vi "内置参数设置.vi"() -> ()   [LabVIEW 2016, in "斯坦道CODMn新电路板.lvlib"]
uses:
  <vilib>/Utility/miscctls.llb/LVPointTypeDef.ctl
panel:
  in  "阀配置:":u8(ring) items=["三通阀", "排阀"]
  in  "AB跨度告警值:":u16
  in  "B值告警上限值:":u16
  in  "B值范围:":u16
  in  "A值告警上限值:":u16
  in  "A值范围:":u16
  in  "是否存在液位检测板:":u16(ring) items=["否", "是"]
  in  "检出限(mg/L):":dbl
  in  "测量精度(mg/L):":dbl
  in  "ILimitDown":dbl
  in  "ILimitUp:":dbl
  in  "K d:":dbl
  in  "K i:":dbl
  in  "K p:":dbl
  in  "加热超时时间:(单位:秒)":dbl
  in  "告警温度:":dbl
  in  "加热温度:  校准参数":dbl
  in  "运行速度:  (修改需要重启)":u16
  in  "偏心轮: 校准参数":dbl
  in  "注射泵加热超时时间(s):":u16
  in  "注射泵保温温度H:":u8
  in  "注射泵\n保温温度L:":u8
  in  "废液通道:":u8
  in  "纯水通道:":u8
  in  "滴定速度:":u16
  in  "出样速度:":u16
  in  "进样速度:":u16
  in  "阀数量:":u8(ring) items=["9通"=9, "12通"=12]
  in  "注射泵型号":u8(ring) items=["TECAN", "润泽"]
  in  "阈值(高→低)(mg/L):":dbl
  in  "阈值(低→高)(mg/L):":dbl
  in  "检测下限(mg/L):":dbl
  in  "检测上限(mg/L):":dbl
  in  "关闭":bool
  in  "保存":bool
  in  "读取":bool
  # "仪器内部参数设置"
  # "~"
  # "~"
  # "~"
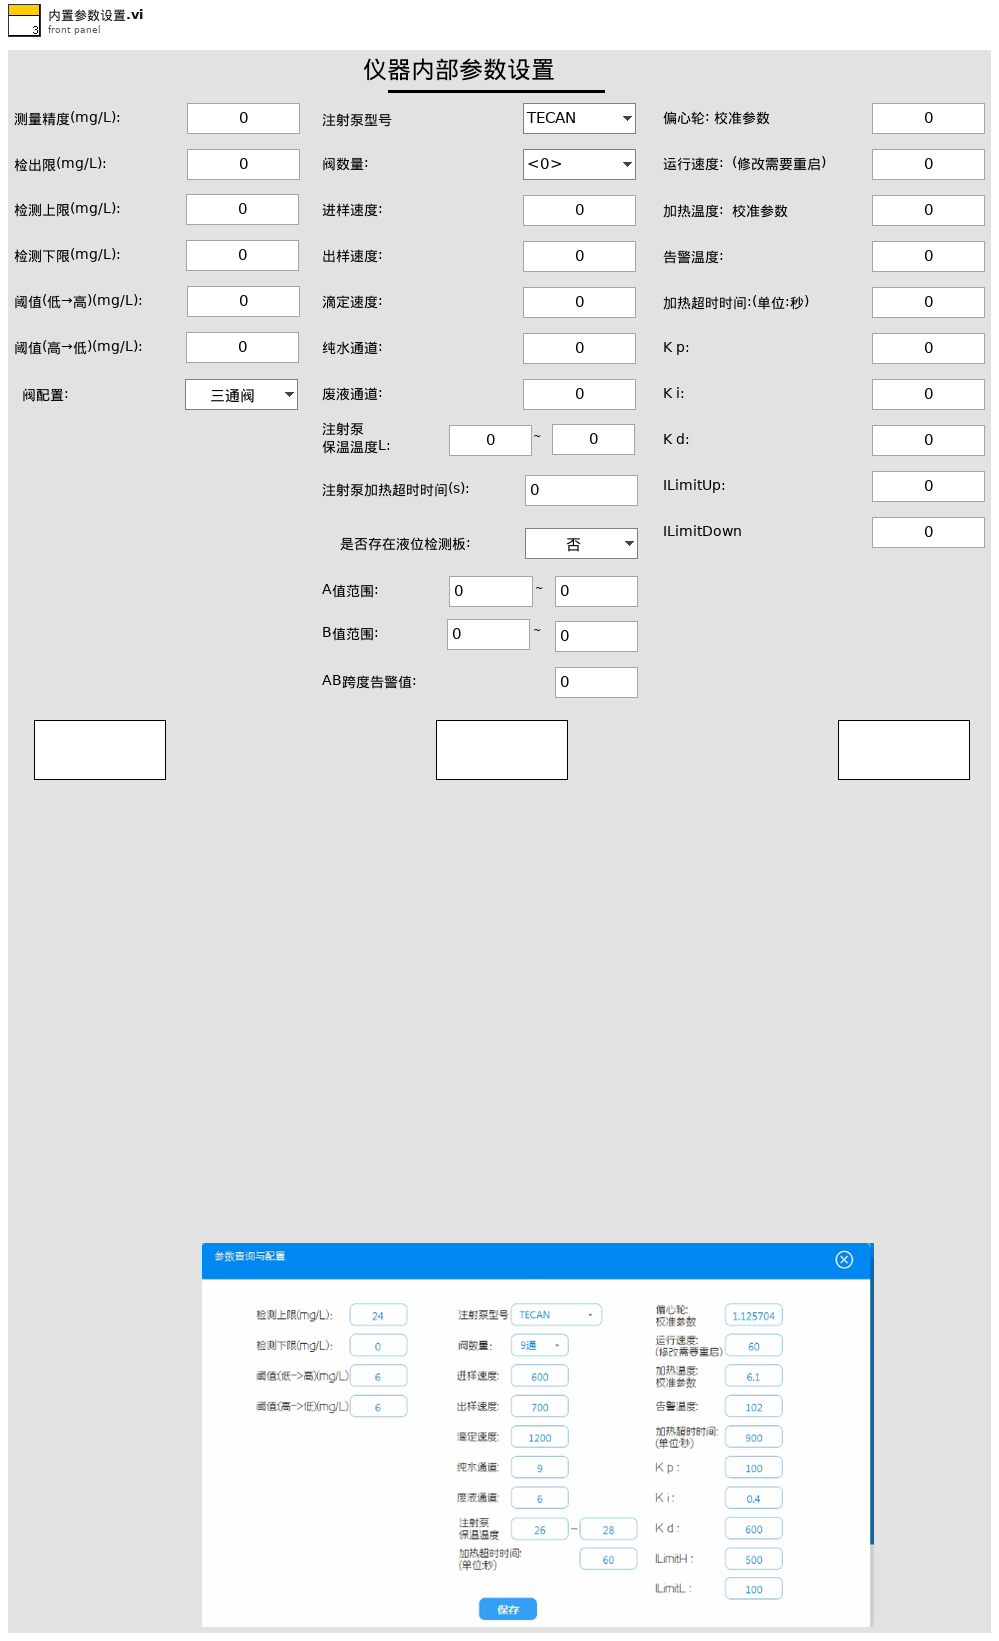
[diagram p1: front panel]
types:
  T1 = typedef "LVPointTypeDef.ctl" = cluster{"Horizontal":i16, "Vertical":i16}
  T2 = cluster{"偏心轮校准参数":dbl, "运行速度(修改需要重启)":u16, "加热温度(校准参数) ":dbl, "告警温度":dbl, "加热超时时间:(单位/秒)":dbl, "K p":dbl, "K i":dbl, "K d":dbl, "ILimitUp":dbl, "ILimitDown":dbl}
  T3 = cluster{"泵类型":u8, "阀数量":u8, "纯水通道":u8, "废液通道":u8, "进样速度":u16, "出样速度":u16, "滴定速度":u16, "注射泵保温温度L":u8, "注射泵保温温度H":u8, "注射泵加热超时时间":u16, "是否存在液位检测板":u16, "A值告警下限值":u16, "A值告警上限值":u16, "B值告警下限值":u16, "B值告警上限值":u16, "AB跨度告警值":u16, "阀配置:":u8}
  T4 = cluster{"检出限":dbl, "测量精度":dbl, "上限":dbl, "下限":dbl, "阈值（低->高）":dbl, "阈值（高->低）":dbl}
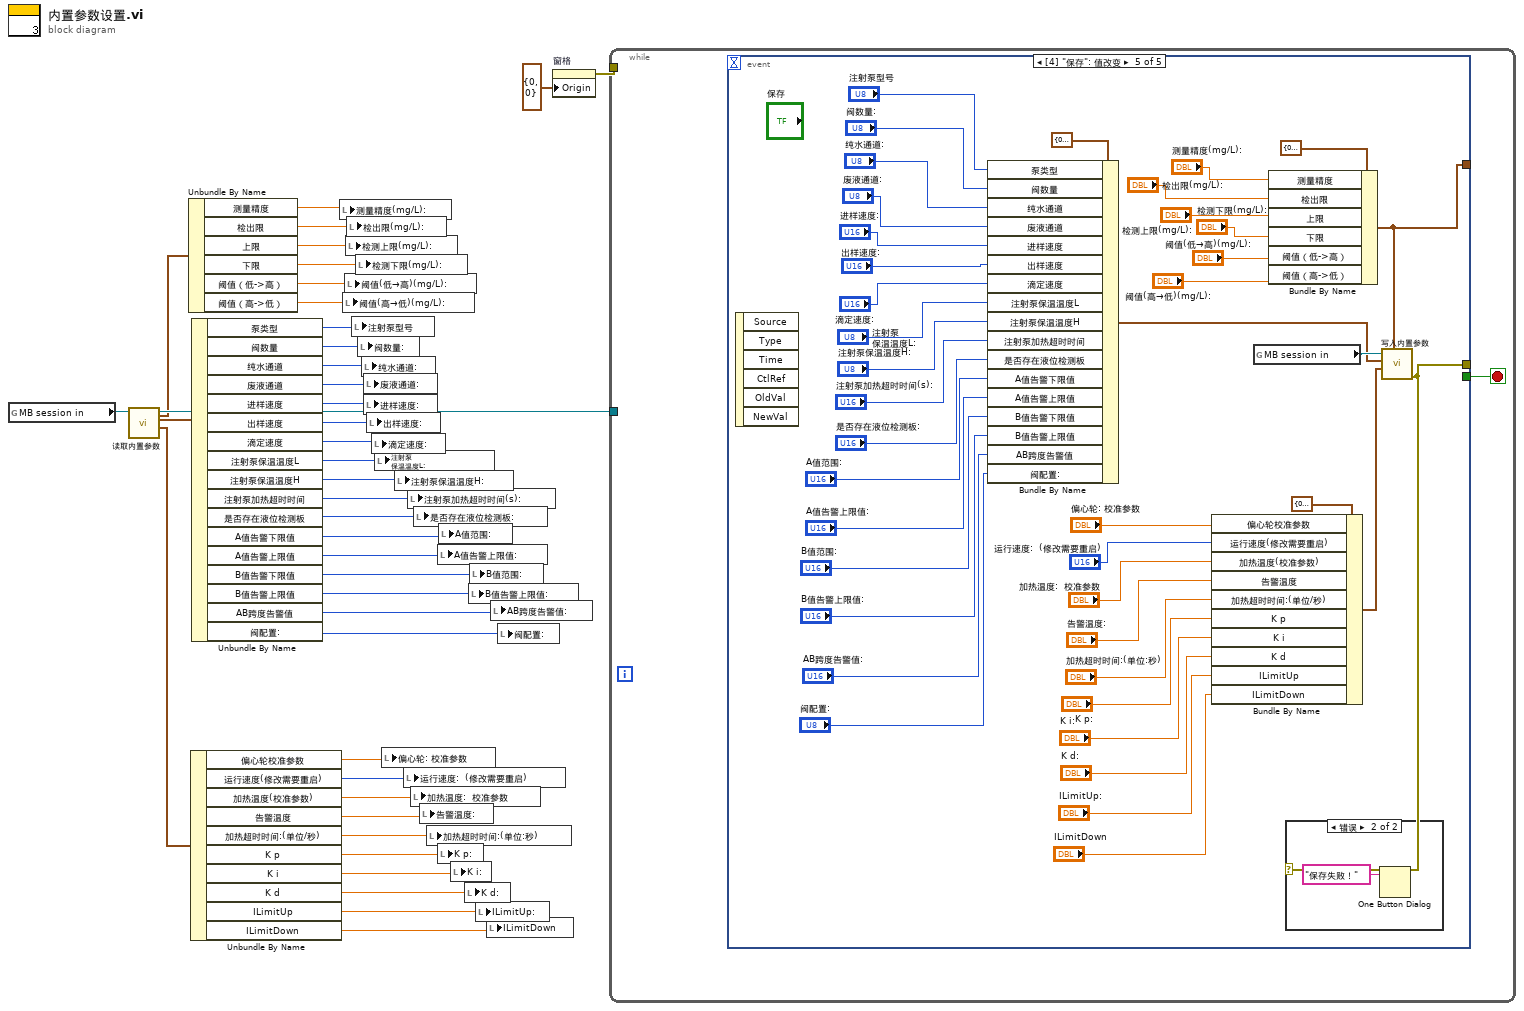
[diagram p0: block diagram]
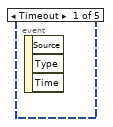
[diagram p2: hidden frame]
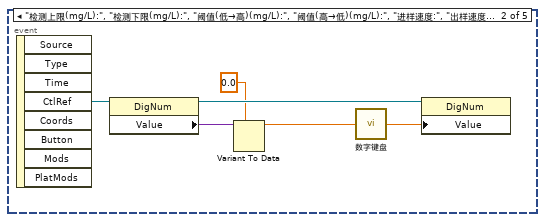
[diagram p3: hidden frame]
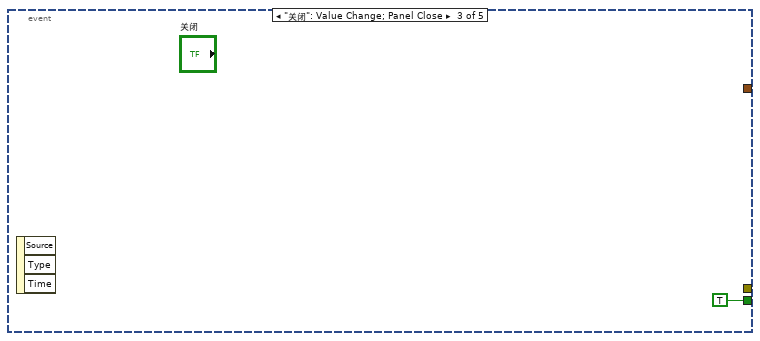
[diagram p4: hidden frame]
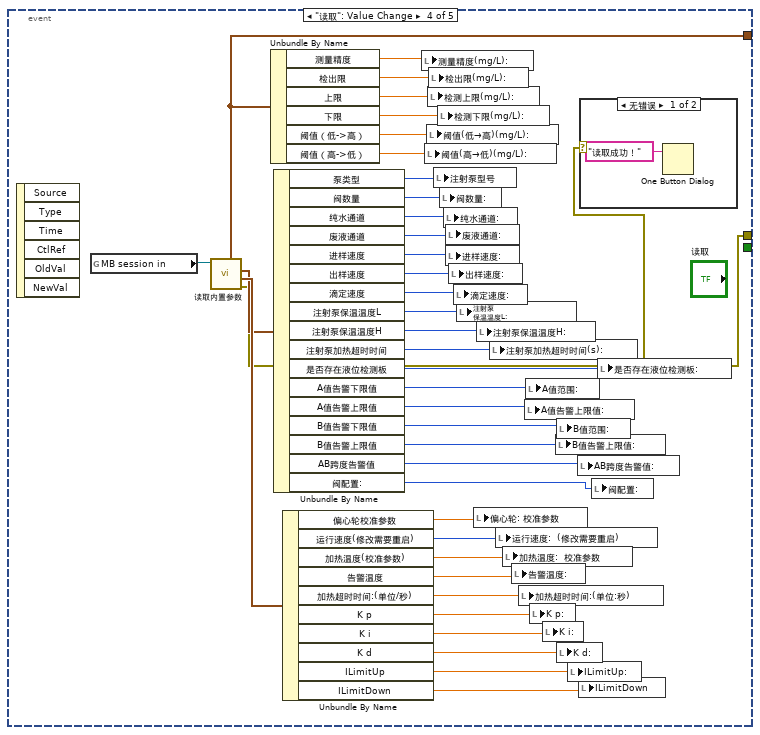
[diagram p5: hidden frame]
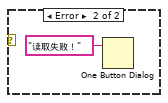
[diagram p6: hidden frame]
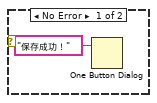
[diagram p7: hidden frame]
diagram:
  n1 = global read "VARCODMn全局变量.vi" "MB session in"() -> (w38:refnum<class "MB_Master.lvclass">)
  n2 = call "读取内置参数.vi"("MB session in"=w38) -> ("float"=w35:T2, "外设配置"=w36:T3, "MB session out"=w37:refnum<class "MB_Master.lvclass">, "量程参数读取"=w1:T4)  [unwired: 6 in, 1 out]
  n3 = Unbundle By Name(w1) -> ("测量精度"=w34:dbl, "检出限"=w33:dbl, "上限"=w32:dbl, "下限"=w31:dbl, "阈值（低->高）"=w30:dbl, "阈值（高->低）"=w29:dbl)
  n4 = Unbundle By Name(w35) -> ("偏心轮校准参数"=w18:dbl, "运行速度(修改需要重启)"=w17:u16, "加热温度(校准参数)"=w16:dbl, "告警温度"=w15:dbl, "加热超时时间:(单位/秒)"=w14:dbl, "K p"=w13:dbl, "K i"=w12:dbl, "K d"=w11:dbl, "ILimitUp"=w10:dbl, "ILimitDown"=w9:dbl)
  n5 = Unbundle By Name(w36) -> ("泵类型"=w28:u8, "阀数量"=w27:u8, "纯水通道"=w26:u8, "废液通道"=w25:u8, "进样速度"=w24:u16, "出样速度"=w23:u16, "滴定速度"=w22:u16, "注射泵保温温度L"=w21:u8, "注射泵保温温度H"=w20:u8, "注射泵加热超时时间"=w19:u16, "是否存在液位检测板"=w8:u16, "A值告警下限值"=w7:u16, "A值告警上限值"=w6:u16, "B值告警下限值"=w5:u16, "B值告警上限值"=w4:u16, "AB跨度告警值"=w3:u16, "阀配置:"=w2:u8)
  n6 = local write "测量精度(mg/L):"(w34) -> ()
  n7 = local write "阈值(高→低)(mg/L):"(w29) -> ()
  n8 = local write "阈值(低→高)(mg/L):"(w30) -> ()
  n9 = local write "检测上限(mg/L):"(w32) -> ()
  n10 = local write "检出限(mg/L):"(w33) -> ()
  n11 = local write "注射泵型号"(w28) -> ()
  n12 = local write "检测下限(mg/L):"(w31) -> ()
  n13 = local write "阀数量:"(w27) -> ()
  n14 = local write "纯水通道:"(w26) -> ()
  n15 = local write "废液通道:"(w25) -> ()
  n16 = local write "进样速度:"(w24) -> ()
  n17 = local write "出样速度:"(w23) -> ()
  n18 = local write "滴定速度:"(w22) -> ()
  n19 = local write "注射泵\n保温温度L:"(w21) -> ()
  n20 = local write "偏心轮: 校准参数"(w18) -> ()
  n21 = local write "注射泵保温温度H:"(w20) -> ()
  n22 = local write "运行速度:  (修改需要重启)"(w17) -> ()
  n23 = local write "注射泵加热超时时间(s):"(w19) -> ()
  n24 = local write "加热温度:  校准参数"(w16) -> ()
  n25 = local write "是否存在液位检测板:"(w8) -> ()
  n26 = local write "告警温度:"(w15) -> ()
  n27 = local write "加热超时时间:(单位:秒)"(w14) -> ()
  n28 = local write "A值告警上限值:"(w6) -> ()
  n29 = local write "K p:"(w13) -> ()
  n30 = local write "A值范围:"(w7) -> ()
  n31 = local write "K i:"(w12) -> ()
  n32 = local write "K d:"(w11) -> ()
  n33 = local write "B值告警上限值:"(w4) -> ()
  n34 = local write "B值范围:"(w5) -> ()
  n35 = local write "ILimitUp:"(w10) -> ()
  n36 = local write "ILimitDown"(w9) -> ()
  n37 = local write "AB跨度告警值:"(w3) -> ()
  n38 = local write "阀配置:"(w2) -> ()
  n39 = property on="窗格" class="Pane"("Origin"=T1 {"Horizontal"=0, "Vertical"=0} ("原点")) -> (error out=w39:errorcluster)  [unwired: 2 in, 1 out]
  n40 = while {
    tunnel: w39 -> [_]
    tunnel: w37 -> [_]
    stop <- w41 stop-if-true
    n41 = event shown="[4] \"保存\": 值改变" {
      selector: _ -> [_ _ _ _ _]
      dyn-events: _ -> [_ _ _ _ _]
      timeout: _ -> [_ _ _ _ _]
      tunnel: [_ _ TRUE _ _] -> w41
      tunnel: [_ _ _ w57 w100] -> _
      tunnel: [_ _ _ w49 w89] -> _
      event Timeout {
        n42 = event-data() -> ()  [unwired: 1 in, 3 out]
      }
      event "检测上限(mg/L):", "检测下限(mg/L):", "阈值(低→高)(mg/L):", "阈值(高→低)(mg/L):", "进样速度:", "出样速度:", "滴定速度:", "纯水通道:", "废液通道:", "注射泵\n保温温度L:", "注射泵保温温度H:", "注射泵加热超时时间(s):", "偏心轮: 校准参数", "运行速度:  (修改需要重启)", "告警温度:", "加热温度:  校准参数", "K p:", "K i:", "K d:", "ILimitUp:", "ILimitDown", "测量精度(mg/L):", "检出限(mg/L):", "A值范围:", "A值告警上限值:", "B值范围:", "B值告警上限值:", "AB跨度告警值:": Mouse Down {
        n43 = event-data() -> ("CtlRef"=w47:refnum<vi>)  [unwired: 1 in, 7 out]
        n44 = property class="DigNum"(reference=w47) -> (reference out=w46:refnum<vi>, "Value"=w44:variant)  [unwired: 1 in, 1 out]
        n45 = Variant To Data(type=0.0 ("OldNumber"), Variant=w44) -> (data=w42:dbl)  [unwired: 1 in, 1 out]
        n46 = call "数字键盘.vi"("OldNumber"=w42) -> ("NewNumber"=w45:dbl)
        n47 = property class="DigNum"(reference=w46, "Value"=w45) -> ()  [unwired: 1 in, 2 out]
      }
      event "关闭": Value Change; Panel Close {
        n48 = event-data() -> ()  [unwired: 1 in, 3 out]
      }
      event "读取": Value Change {
        n49 = event-data() -> ()  [unwired: 1 in, 6 out]
        n50 = global read "VARCODMn全局变量.vi" "MB session in"() -> (w58:refnum<class "MB_Master.lvclass">)
        n51 = call "读取内置参数.vi"("MB session in"=w58) -> ("error out"=w57:errorcluster, "float"=w60:T2, "外设配置"=w59:T3, "量程参数读取"=w49:T4)  [unwired: 6 in, 1 out]
        n52 = Unbundle By Name(w49) -> ("测量精度"=w61:dbl, "检出限"=w62:dbl, "上限"=w63:dbl, "下限"=w64:dbl, "阈值（低->高）"=w65:dbl, "阈值（高->低）"=w66:dbl)
        n53 = Unbundle By Name(w59) -> ("泵类型"=w67:u8, "阀数量"=w68:u8, "纯水通道"=w69:u8, "废液通道"=w70:u8, "进样速度"=w71:u16, "出样速度"=w72:u16, "滴定速度"=w73:u16, "注射泵保温温度L"=w74:u8, "注射泵保温温度H"=w75:u8, "注射泵加热超时时间"=w76:u16, "是否存在液位检测板"=w56:u16, "A值告警下限值"=w55:u16, "A值告警上限值"=w54:u16, "B值告警下限值"=w53:u16, "B值告警上限值"=w52:u16, "AB跨度告警值"=w51:u16, "阀配置:"=w50:u8)
        n54 = Unbundle By Name(w60) -> ("偏心轮校准参数"=w77:dbl, "运行速度(修改需要重启)"=w78:u16, "加热温度(校准参数)"=w79:dbl, "告警温度"=w80:dbl, "加热超时时间:(单位/秒)"=w81:dbl, "K p"=w82:dbl, "K i"=w83:dbl, "K d"=w84:dbl, "ILimitUp"=w85:dbl, "ILimitDown"=w86:dbl)
        n55 = local write "测量精度(mg/L):"(w61) -> ()
        n56 = local write "阈值(高→低)(mg/L):"(w66) -> ()
        n57 = local write "阈值(低→高)(mg/L):"(w65) -> ()
        n58 = local write "检测上限(mg/L):"(w63) -> ()
        n59 = local write "检出限(mg/L):"(w62) -> ()
        n60 = local write "注射泵型号"(w67) -> ()
        n61 = local write "检测下限(mg/L):"(w64) -> ()
        n62 = local write "阀数量:"(w68) -> ()
        n63 = local write "纯水通道:"(w69) -> ()
        n64 = local write "废液通道:"(w70) -> ()
        n65 = local write "进样速度:"(w71) -> ()
        n66 = local write "出样速度:"(w72) -> ()
        n67 = local write "滴定速度:"(w73) -> ()
        n68 = local write "注射泵\n保温温度L:"(w74) -> ()
        n69 = local write "偏心轮: 校准参数"(w77) -> ()
        n70 = local write "注射泵保温温度H:"(w75) -> ()
        n71 = local write "注射泵加热超时时间(s):"(w76) -> ()
        n72 = local write "运行速度:  (修改需要重启)"(w78) -> ()
        n73 = local write "加热温度:  校准参数"(w79) -> ()
        n74 = local write "告警温度:"(w80) -> ()
        n75 = local write "加热超时时间:(单位:秒)"(w81) -> ()
        n76 = local write "A值告警上限值:"(w54) -> ()
        n77 = local write "A值范围:"(w55) -> ()
        n78 = local write "K p:"(w82) -> ()
        n79 = local write "K i:"(w83) -> ()
        n80 = local write "B值告警上限值:"(w52) -> ()
        n81 = local write "B值范围:"(w53) -> ()
        n82 = local write "K d:"(w84) -> ()
        n83 = local write "ILimitUp:"(w85) -> ()
        n84 = local write "AB跨度告警值:"(w51) -> ()
        n85 = local write "ILimitDown"(w86) -> ()
        n86 = case shown="无错误" w57 {
          frame No Error {
            n87 = One Button Dialog(message="读取成功！" ("消息")) -> ()  [unwired: 1 in, 1 out]
          }
          frame Error {
            n88 = One Button Dialog(message="读取失败！" ("消息")) -> ()  [unwired: 1 in, 1 out]
          }
        }
        n89 = local write "阀配置:"(w50) -> ()
        n90 = local write "是否存在液位检测板:"(w56) -> ()
      }
      event "保存": Value Change {
        n91 = event-data() -> ()  [unwired: 1 in, 6 out]
        n92 = Bundle By Name(cluster=T3 {"泵类型"=0, "阀数量"=0, "纯水通道"=0, "废液通道"=0, "进样速度"=0, "出样速度"=0, "滴定速度"=0, "注射泵保温温度L"=0, "注射泵保温温度H"=0, "注射泵加热超时时间"=0, "是否存在液位检测板"=0, "A值告警下限值"=0, "A值告警上限值"=0, "B值告警下限值"=0, "B值告警上限值"=0, "AB跨度告警值"=0, "阀配置:"=0} ("外设配置"), "泵类型"="注射泵型号", "阀数量"="阀数量:", "纯水通道"="纯水通道:", "废液通道"="废液通道:", "进样速度"="进样速度:", "出样速度"="出样速度:", "滴定速度"="滴定速度:", "注射泵保温温度L"="注射泵\n保温温度L:", "注射泵保温温度H"="注射泵保温温度H:", "注射泵加热超时时间"="注射泵加热超时时间(s):", "是否存在液位检测板"="是否存在液位检测板:", "A值告警下限值"="A值范围:", "A值告警上限值"="A值告警上限值:", "B值告警下限值"="B值范围:", "B值告警上限值"="B值告警上限值:", "AB跨度告警值"="AB跨度告警值:", "阀配置:"="阀配置:") -> (w93:T3)
        n93 = Bundle By Name(cluster=T2 {"偏心轮校准参数"=0.0, "运行速度(修改需要重启)"=0, "加热温度(校准参数) "=0.0, "告警温度"=0.0, "加热超时时间:(单位/秒)"=0.0, "K p"=0.0, "K i"=0.0, "K d"=0.0, "ILimitUp"=0.0, "ILimitDown"=0.0} ("float"), "偏心轮校准参数"="偏心轮: 校准参数", "运行速度(修改需要重启)"="运行速度:  (修改需要重启)", "加热温度(校准参数)"="加热温度:  校准参数", "告警温度"="告警温度:", "加热超时时间:(单位/秒)"="加热超时时间:(单位:秒)", "K p"="K p:", "K i"="K i:", "K d"="K d:", "ILimitUp"="ILimitUp:", "ILimitDown"="ILimitDown") -> (w101:T2)
        n94 = global read "VARCODMn全局变量.vi" "MB session in"() -> (w129:refnum<class "MB_Master.lvclass">)
        n95 = Bundle By Name(cluster=T4 {"检出限"=0.0, "测量精度"=0.0, "上限"=0.0, "下限"=0.0, "阈值（低->高）"=0.0, "阈值（高->低）"=0.0} ("量程参数读取"), "测量精度"="测量精度(mg/L):", "检出限"="检出限(mg/L):", "上限"="检测上限(mg/L):", "下限"="检测下限(mg/L):", "阈值（低->高）"="阈值(低→高)(mg/L):", "阈值（高->低）"="阈值(高→低)(mg/L):") -> (w89:T4)
        n96 = call "写入内置参数.vi"("量程参数读取"=w89, "float"=w101, "外设配置"=w93, "MB session in"=w129) -> ("error out"=w100:errorcluster)  [unwired: 6 in, 1 out]
        n97 = case shown="错误" w100 {
          frame No Error {
            n98 = One Button Dialog(message="保存成功！" ("消息")) -> ()  [unwired: 1 in, 1 out]
          }
          frame Error {
            n99 = One Button Dialog(message="保存失败！" ("消息")) -> ()  [unwired: 1 in, 1 out]
          }
        }
      }
    }
  }
